vi "Get Target.vi"(6 "Axis":T1, 8 "error in (no error)":errorcluster, 11 "Instrument.VRM in":refnum<class "Instrument.OxfordVRM.lvclass">) -> (0 "error out":errorcluster, 1 "Target Field Rate (T/min)":dbl, 2 "Target Field (T)":dbl, 3 "Instrument.VRM out":refnum<class "Instrument.OxfordVRM.lvclass">)   [LabVIEW 2016, in "Instrument.OxfordVRM.lvclass"]
uses:
  Instrument.OxfordVRM.lvclass
  <userlib>/LevyLab/Levylab Instruments/Instrument Types/Cryostat/Typedefs/VRM Magnet Axis--Enum.ctl
  Typedefs/Instrument.VRM.Commands-enum.ctl
  Typedefs/VRM Targets--Cluster.ctl
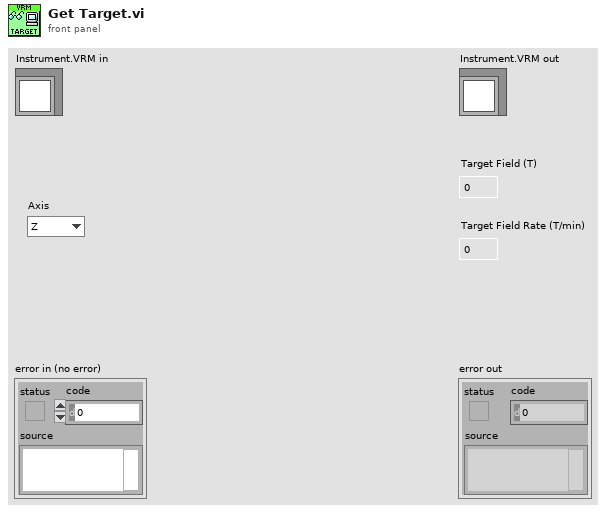
[diagram p1: front panel]
types:
  T1 = typedef "Instrument.OxfordVRM.lvclass/VRM Magnet Axis--Enum.ctl" = enum16{"Z", "X", "Y", "ALL"}
  T2 = typedef "Instrument.OxfordVRM.lvclass/VRM Targets--Cluster.ctl" = cluster{"Field (T)":dbl, "Field Rate (T/min)":dbl, "Axis":T1}
  T3 = typedef "Instrument.OxfordVRM.lvclass/Instrument.VRM.Commands-enum.ctl" = enum16{"setAction", "setTarget", "setMagnetField", "getStatus", "getTarget", "getMagnetField"}
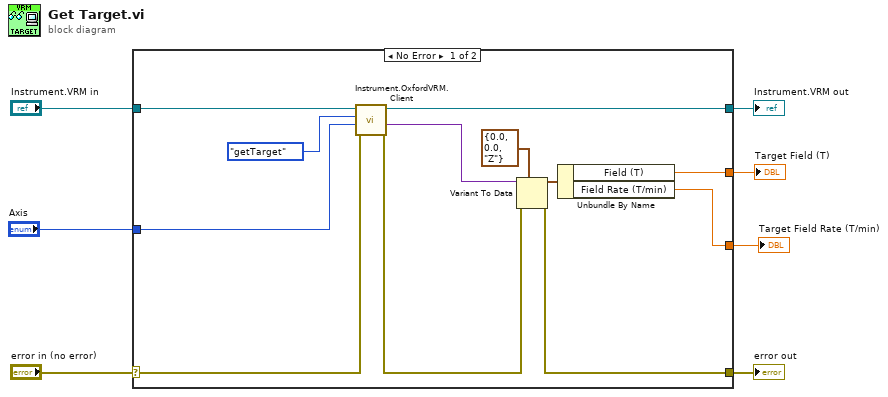
[diagram p0: block diagram]
diagram:
  n1 = case shown="No Error" "error in (no error)" {
    selector: "error in (no error)" -> [w18 w21]
    tunnel: [w16 w21] -> w6
    tunnel: [w10 w20] -> w4
    tunnel: "Instrument.VRM in" -> [w11 w20]
    tunnel: [w13 _] -> w3
    tunnel: [w12 _] -> w2
    tunnel: "Axis" -> [w8 _]
    frame No Error {
      n2 = call "Instrument.OxfordVRM.Client.vi"("error in (no error)"=w18, "Data"=w8, "Commands"=Instrument.VRM.Commands-enum."getTarget", "Instrument.VRM in"=w11) -> ("error out"=w17:errorcluster, "Data out"=w9:variant, "Instrument.VRM out"=w10:refnum<class "Instrument.OxfordVRM.lvclass">)  [unwired: 5 in]
      n3 = Variant To Data(error in=w17, type=T2 {"Field (T)"=0.0, "Field Rate (T/min)"=0.0, "Axis"=enum."Z"} ("Target"), Variant=w9) -> (data=w14:T2, error out=w16:errorcluster)
      n4 = Unbundle By Name(w14) -> ("Field (T)"=w13:dbl, "Field Rate (T/min)"=w12:dbl)
    }
    frame Error {
    }
  }
  "error out" <- w6
  "Instrument.VRM out" <- w4
  "Target Field (T)" <- w3
  "Target Field Rate (T/min)" <- w2
